vi "Adresse Geraet Kennung.vi"(8 "error in (no error)":errorcluster caption="Fehler (Eingang, kein Fehler)", 11 "Schneider Steuerung PNS Eingang":refnum<class "Schneider Steuerung PNS.lvclass">) -> (0 "error out":errorcluster caption="Fehler (Ausgang)", 2 "Adressen":cluster{i32[][], i32}, 3 "Schneider Steuerung PNS Ausgang":refnum<class "Schneider Steuerung PNS.lvclass">)   [LabVIEW 2020, in "Schneider Steuerung PNS.lvclass"]
uses:
  Schneider Steuerung PNS.lvclass
  D:/Software/LabVIEW/LV2020/Compact_LP/LP und Compact Standardprogramm/ObjektKlassen/Steuerung PNS/Steuerung PNS.lvclass
  AdressIndex.ctl
  Steuerung PNS.lvclass
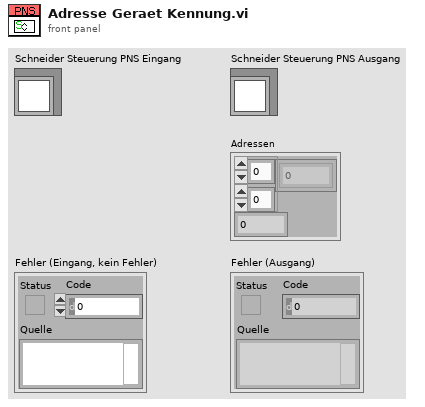
[diagram p1: front panel]
types:
  T1 = typedef "Steuerung PNS.lvclass/AdressIndex.ctl" = cluster{"Index":i32, "Index 2":i32, "Länge2":i32, "\nAnzahl":i32}
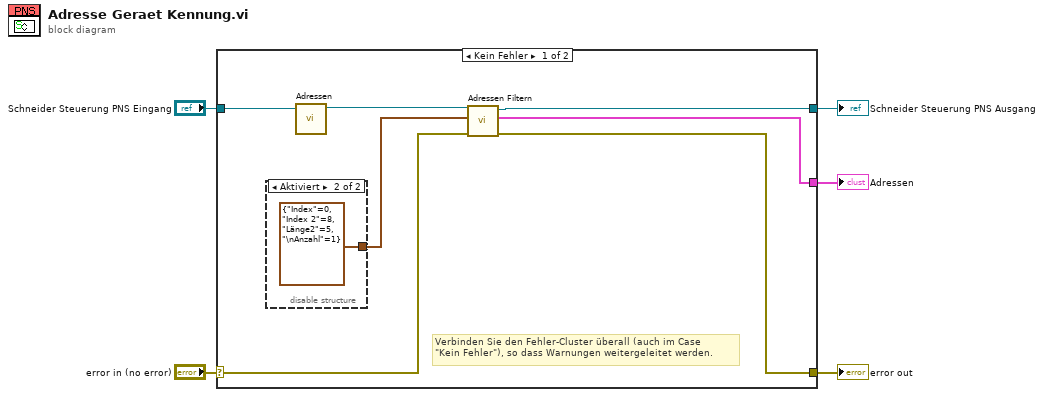
[diagram p0: block diagram]
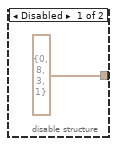
[diagram p2: hidden frame]
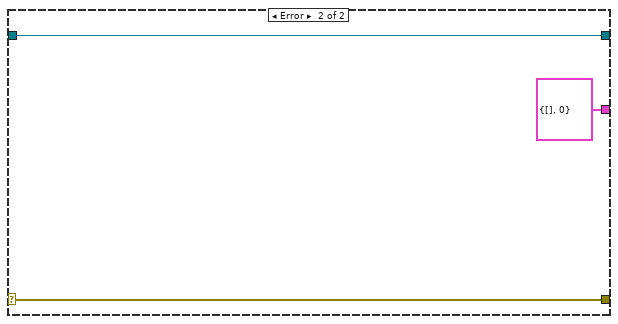
[diagram p3: hidden frame]
diagram:
  n1 = case shown="Kein Fehler" "error in (no error)" {
    selector: "error in (no error)" -> [w10 w17]
    tunnel: [w7 w17] -> w4
    tunnel: [w8 w16] -> w2
    tunnel: "Schneider Steuerung PNS Eingang" -> [w12 w16]
    tunnel: [w6 cluster{i32[][], i32} {[], 0} ("Adressen")] -> w1
    frame No Error {
      # "Verbinden Sie den Fehler-Cluster überall (auch im Case\n\"Kein Fehler\"), so dass Warnungen weitergeleitet werden."
      n2 = disable-structure shown="Aktiviert" {
        disable-tunnel: [T1 {"Index"=0, "Index 2"=8, "Länge2"=3, "\nAnzahl"=1} ("AdressIndex") T1 {"Index"=0, "Index 2"=8, "Länge2"=5, "\nAnzahl"=1} ("AdressIndex")] -> w9
        frame Disabled {
        }
        frame Enabled {
        }
      }
      n3 = call-dynamic "Adressen.vi"("Schneider Steuerung PNS Eingang"=w12) -> ("Schneider Steuerung PNS Ausgang"=w11:refnum<class "Schneider Steuerung PNS.lvclass">)  [unwired: 8 in, 2 out]
      n4 = call "Adressen Filtern.vi"("error in (no error)"=w10, "AdressIndex"=w9, "Steuerung PNS Eingang"=w11) -> ("error out"=w7:errorcluster, "Adressen"=w6:cluster{i32[][], i32}, "Steuerung PNS Ausgang"=w8:refnum<class "Schneider Steuerung PNS.lvclass">)  [unwired: 6 in]
    }
    frame Error {
    }
  }
  "error out" <- w4
  "Schneider Steuerung PNS Ausgang" <- w2
  "Adressen" <- w1
